vi "H-MEDI ReCommunicationPopup.vi"(8 "에러 입력(에러 없음)":errorcluster, 11 "inputResourceName":refnum<visa-resource-name>="COM3") -> (0 "error out":errorcluster caption="에러 출력", 3 "returnResourceName":refnum<visa-resource-name>="COM3")   [LabVIEW 2019]
doc: "30"
uses:
  <vilib>/Utility/miscctls.llb/LVPointTypeDef.ctl
  <vilib>/Instr/_visa.llb/VISA Configure Serial Port (Instr).vi
panel:
  in  "userContolResourceName":refnum<visa-resource-name>="COM3"
  in  "다음":bool
  out "연결 상태 확인":bool
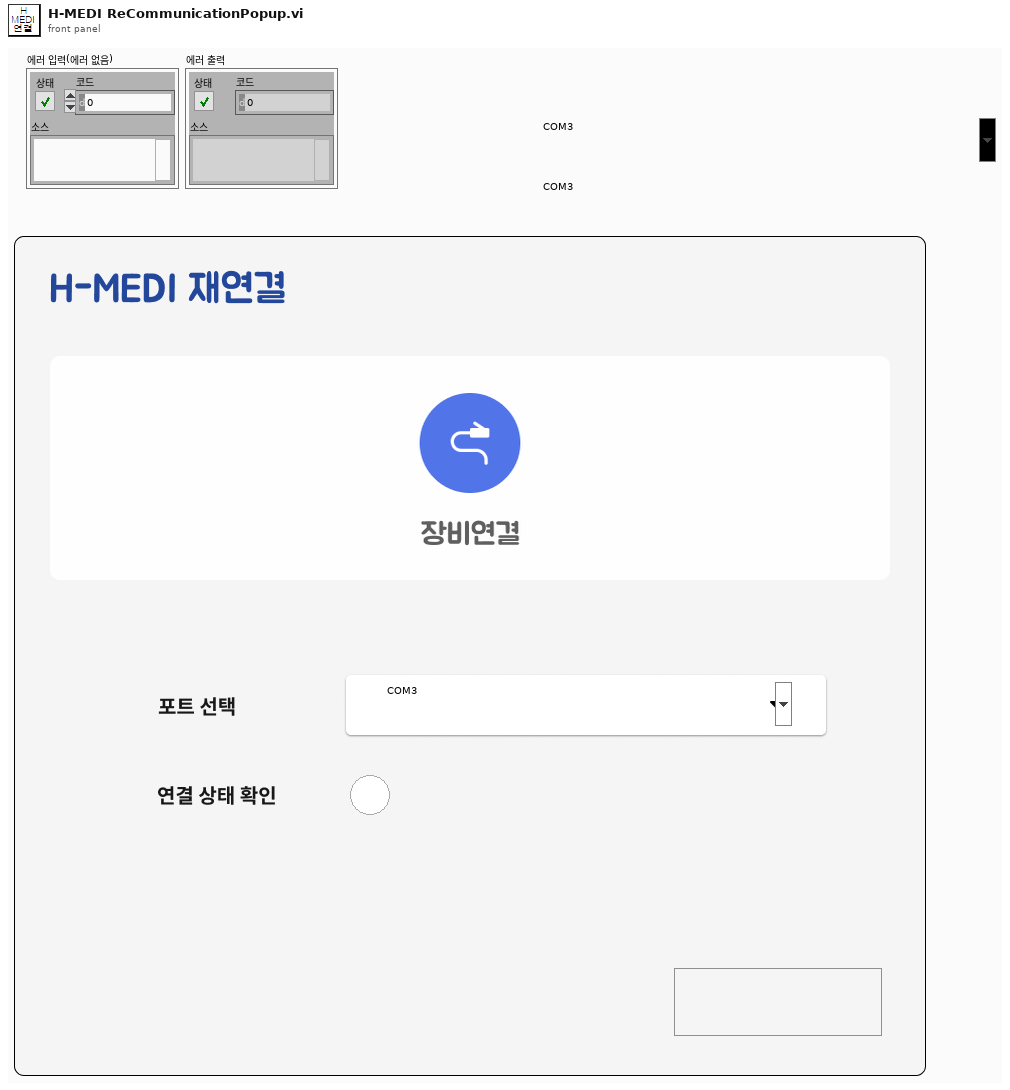
[diagram p1: front panel]
types:
  T1 = typedef "LVPointTypeDef.ctl" = cluster{"Horizontal":i16, "Vertical":i16}
  T2 = cluster{"baud rate (9600)":u32, "flow control (0:none)":u16, "VISA resource name 2":refnum<visa-resource-name>, "termination char\n(0xA = '\\n' = LF) ":u8, "data bits (8)":u16, "parity (0:none)":enum16{"None", "Odd", "Even", "Mark", "Space"}, "timeout (10sec)":u32, "Enable Termination\nChar (T)":bool, "stop bits (10: 1 bit)":u16}
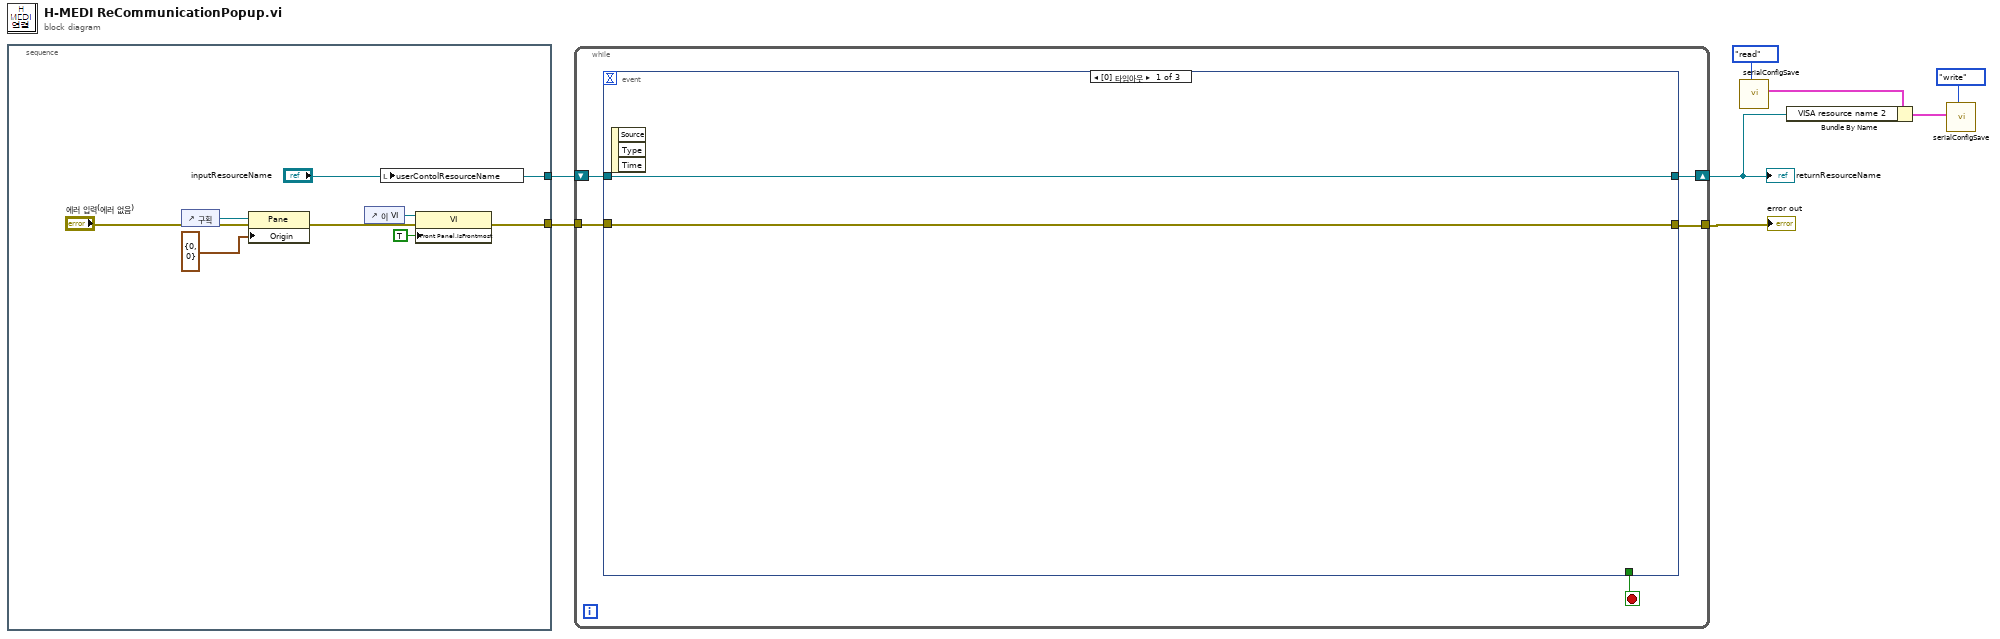
[diagram p0: block diagram]
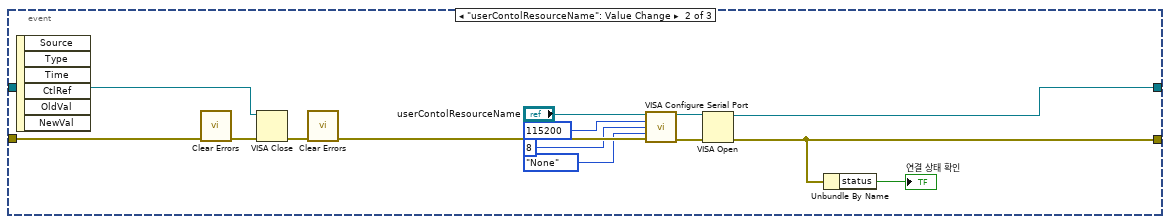
[diagram p2: hidden frame]
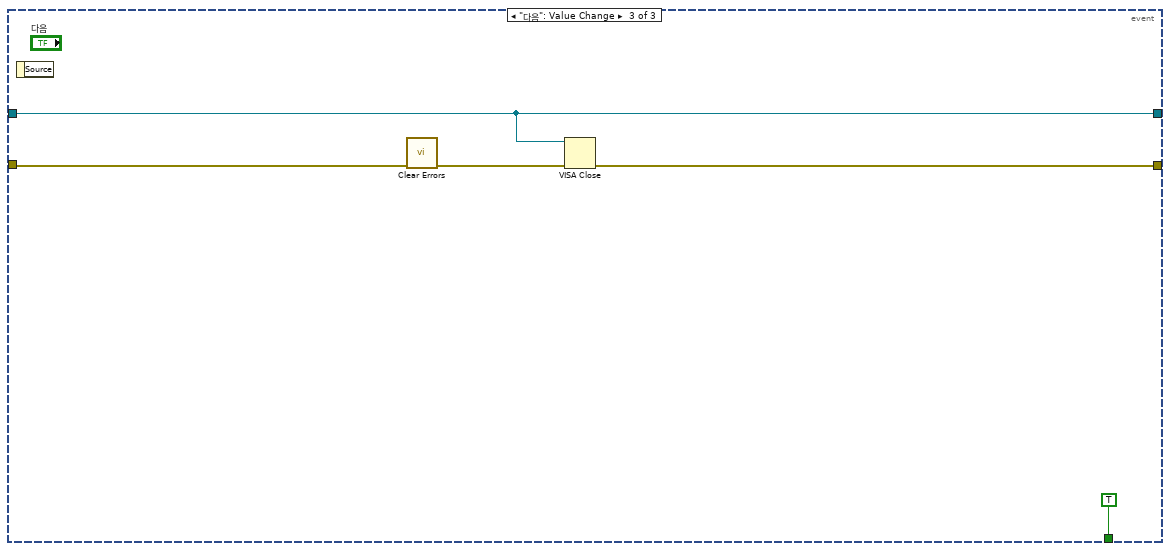
[diagram p3: hidden frame]
diagram:
  n1 = stacked-sequence {
    tunnel: [w11] -> w8
    tunnel: ["inputResourceName"] -> w7
    frame #0 {
      n2 = control-ref of="구획"() -> (w14:refnum<vi>)
      n3 = property class="Pane"(reference=w14, error in="에러 입력(에러 없음)", "Origin"=T1 {"Horizontal"=0, "Vertical"=0} ("원점")) -> (error out=w12:errorcluster)  [unwired: 1 out]
      n4 = control-ref of="이 VI"() -> (w16:refnum<vi>)
      n5 = local write "userContolResourceName"("inputResourceName") -> ()
      n6 = property class="VI"(reference=w16, error in=w12, "Front Panel.IsFrontmost"=TRUE ("프런트패널 윈도우:맨 앞으로")) -> (error out=w11:errorcluster)  [unwired: 1 out]
    }
  }
  n7 = while {
    tunnel: w8 -> [w20]
    shift-right: [w17] -> w2
    shift-left: w7 -> [w19]
    tunnel: [w18] -> w6
    stop <- w21 stop-if-true
    n8 = event shown="[0] 타임아웃" {
      selector: _ -> [_ _ _]
      dyn-events: _ -> [_ _ _]
      timeout: _ -> [_ _ _]
      tunnel: [_ _ TRUE] -> w21
      tunnel: w20 -> [w22 w28 w41]
      tunnel: w19 -> [w23 w27 w38]
      tunnel: [w22 w25 w39] -> w18
      tunnel: [w23 w26 w38] -> w17
      event Timeout {
        n9 = event-data() -> ()  [unwired: 1 in, 3 out]
      }
      event "userContolResourceName": Value Change {
        n10 = event-data() -> ()  [unwired: 1 in, 6 out]
        n11 = call <vilib>:"Clear Errors.vi"("error in (no error)"=w28) -> ("error out"=w37:errorcluster)  [unwired: 5 in, 1 out]
        n12 = VISA Close(VISA resource name=w27, error in (no error)=w37) -> (error out=w36:errorcluster)
        n13 = call <vilib>:"Clear Errors.vi"("error in (no error)"=w36) -> ("error out"=w35:errorcluster)  [unwired: 5 in, 1 out]
        n14 = call-poly "VISA Configure Serial Port"("VISA resource name"="userContolResourceName", "baud rate (9600)"=u32 115200, "data bits (8)"=u16 8, "parity (0:none)"=enum16{"None", "Odd", "Even", "Mark", "Space"}."None", "error in (no error)"=w35) -> ("VISA resource name out"=w29:refnum<visa-resource-name>, "error out"=w30:errorcluster)  [unwired: 9 in]
        n15 = VISA Open(error in (no error)=w30, VISA resource name=w29) -> (VISA resource name=w26:refnum<visa-resource-name>, error out=w25:errorcluster)  [unwired: 3 in]
        n16 = Unbundle By Name(w25) -> ("status"=→"연결 상태 확인":bool)
      }
      event "다음": Value Change {
        n17 = event-data() -> ()  [unwired: 1 in, 1 out]
        n18 = call <vilib>:"Clear Errors.vi"("error in (no error)"=w41) -> ("error out"=w40:errorcluster)  [unwired: 5 in, 1 out]
        n19 = VISA Close(VISA resource name=w38, error in (no error)=w40) -> (error out=w39:errorcluster)
      }
    }
  }
  "error out" <- w6
  "returnResourceName" <- w2
  n20 = call "serialConfigSave.vi"("Ctl"=enum16{"read", "write"}."read") -> ("Reurn"=w3:T2)  [unwired: 10 in]
  n21 = Bundle By Name(cluster=w3, "VISA resource name 2"=w2) -> (w1:T2)
  n22 = call "serialConfigSave.vi"("Ctl"=enum16{"read", "write"}."write", "ViSA Config"=w1) -> ()  [unwired: 9 in, 1 out]
